vi "Destroy.vi"(8 "error in (no error)":errorcluster, 11 "CIF_NIChn_FIFO_DAQ in":refnum<class "CIF_NIChn_FIFO_DAQ_DVR.lvclass">) -> (0 "error out":errorcluster, 3 "CIF_NIChn_FIFO_DAQ out":refnum<class "CIF_NIChn_FIFO_DAQ_DVR.lvclass">)   [LabVIEW 2021, in "CIF_NIChn_FIFO_DAQ_DVR.lvclass"]
uses:
  CIF_NIChn_FIFO_DAQ_DVR.lvclass
  D:/dev/Packages/Channel_Manager/src/CIF_NIChn/NIChn/CIF_NIChn.lvclass
  D:/dev/Packages/Channel_Manager/src/CIFChannels/CIFChannels.lvclass
  NIChn/CIF_NIChn.lvclass/CIF_NIChn.ctl
  CIFChannels/CIFChannels.lvclass/CIFChannels.ctl
  CIF_NIChn_FIFO_DAQ_DVR.lvclass/CIF_NIChn_FIFO_DAQ_DVR.ctl
  ChannelCommon/typedef/Datatype Waveform.ctl
  <vilib>/CIF Foundation/CIF Channels/CIFChannels/SubVIs/CIFServices Fill In Error Info Ex.vi
  <vilib>/CIF Foundation/CIF Channels/CIFChannels/SubVIs/Get dll Path.vi
  <vilib>/CIF Foundation/CIF Utilities/Errors/Append Error Location.vi
  NIChn/CIF_NIChn.lvclass
  <vilib>/CIF Foundation/CIF Channels/CIFChannels/CIFChannelCore.lvlib
  CIFChannels/CIFChannels.lvclass
  ChannelCommon/ChannelCommon.lvlib
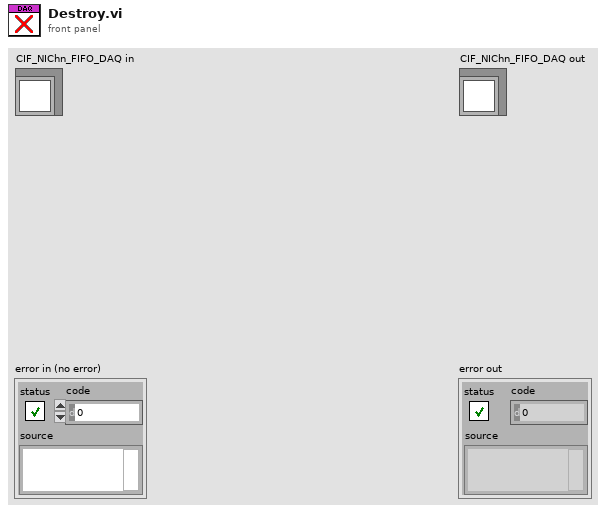
[diagram p1: front panel]
types:
  T1 = typedef "CIFChannels.lvclass/Direction.ctl" = enum16{"Publisher", "Subscriber"}
  T2 = typedef "ChannelCommon.lvlib/Datatype Waveform.ctl" = cluster{"measurement":dbl[], "dT":dbl, "Timestamp":i64, "Read Lock":bool}
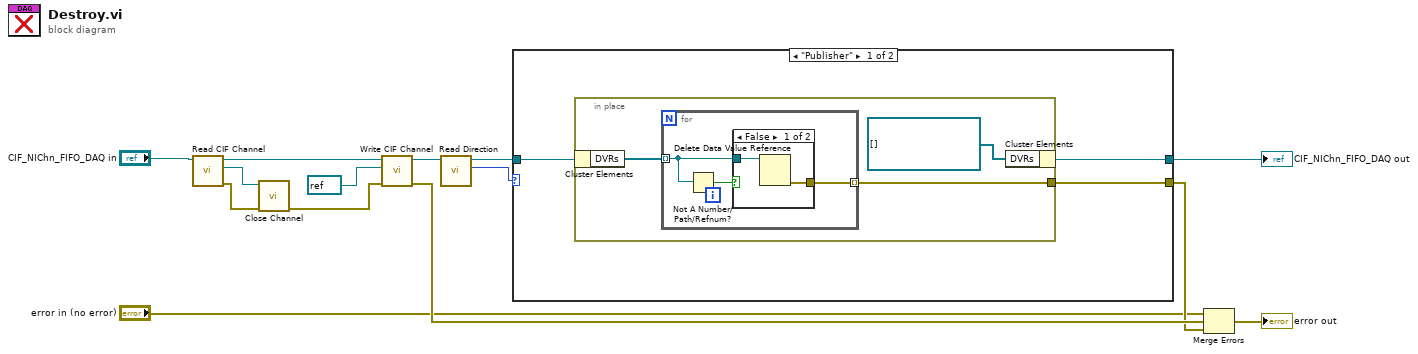
[diagram p0: block diagram]
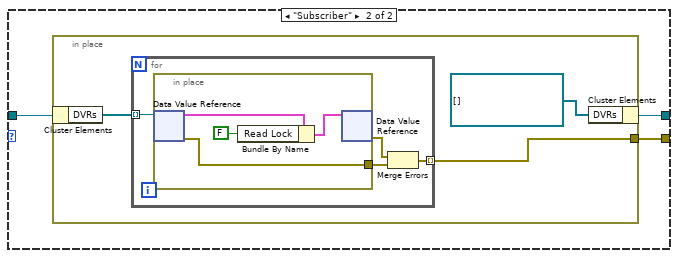
[diagram p3: hidden frame]
diagram:
  n1 = call "Read CIF Channel.vi"("CIFTag in"="CIF_NIChn_FIFO_DAQ in") -> ("error out"=w10:errorcluster, "CIF Channel"=w14:refnum<k21>, "CIFTag out"=w12:refnum<class "CIF_NIChn_FIFO_DAQ_DVR.lvclass">)  [unwired: 8 in]
  n2 = call <vilib>:"Close Channel.vi"("error in"=w10, "CIF Channel"=w14) -> ("error out"=w11:errorcluster)  [unwired: 9 in]
  n3 = call "Write CIF Channel.vi"("error in (no error)"=w11, "CIF Channel"=refnum<k21> refnum, "CIFTag in"=w12) -> ("error out"=w6:errorcluster, "CIFTag out"=w9:refnum<class "CIF_NIChn_FIFO_DAQ_DVR.lvclass">)  [unwired: 7 in]
  n4 = call "Read Direction.vi"("CIFChannels in"=w9) -> ("Direction"=w8:T1, "CIFChannels out"=w7:refnum<class "CIF_NIChn_FIFO_DAQ_DVR.lvclass">)  [unwired: 8 in, 1 out]
  n5 = case shown="\"Publisher\"" w8 {
    tunnel: [w17 w28] -> w1
    tunnel: w7 -> [w16 w27]
    tunnel: [w15 w26] -> w5
    frame "Publisher" {
      n6 = in-place {
        in-place-border: [w18] -> w15
        n7 = in-place-cluster #1(w16) -> ("DVRs"=w20:refnum<data-value>[])
        n8 = for {
          tunnel: w20 -> [w22] mode=indexing
          tunnel: [w23] -> w18 mode=indexing
          n9 = Not A Number/Path/Refnum?(number/path/refnum=w22) -> (NaN/Path/Refnum?=w21:bool)
          n10 = case shown="False" w21 {
            tunnel: [w25 _] -> w23
            tunnel: w22 -> [w24 _]
            frame False {
              n11 = Delete Data Value Reference(data value reference=w24) -> (error out=w25:errorcluster)  [unwired: 1 in, 1 out]
            }
            frame True {
            }
          }
        }
        n12 = in-place-cluster #1("DVRs"=refnum<data-value>[] []) -> (w17:refnum<class "CIF_NIChn_FIFO_DAQ_DVR.lvclass">)
      }
    }
    frame "Subscriber" {
      n13 = in-place {
        in-place-border: [w29] -> w26
        n14 = in-place-cluster #2(w27) -> ("DVRs"=w30:refnum<data-value>[])
        n15 = for {
          tunnel: w30 -> [w35] mode=indexing
          tunnel: [w32] -> w29 mode=indexing
          n16 = in-place {
            in-place-border: [w39] -> w34
            n17 = in-place-dvr #3(w35) -> (w38:T2, w39:errorcluster)
            n18 = Bundle By Name(cluster=w38, "Read Lock"=FALSE) -> (w37:T2)
            n19 = in-place-dvr #3(w37) -> (w33:errorcluster)  [unwired: 1 out]
          }
          n20 = Merge Errors(w33, w34) -> (w32:errorcluster)
        }
        n21 = in-place-cluster #2("DVRs"=refnum<data-value>[] []) -> (w28:refnum<class "CIF_NIChn_FIFO_DAQ_DVR.lvclass">)
      }
    }
  }
  "CIF_NIChn_FIFO_DAQ out" <- w1
  n22 = Merge Errors("error in (no error)", w6, w5) -> (→"error out":errorcluster)
